vi "D_Array_to_Window.vi"(7 "Window Number (0...15)":i32, 8 "error in (no error)":errorcluster, 11 "Image Pixels (U8)":u8[][](array[numeric])) -> (0 "error out":errorcluster)   [LabVIEW 2015]
uses:
  SLM_Control_VI_source/Image_Control.dll
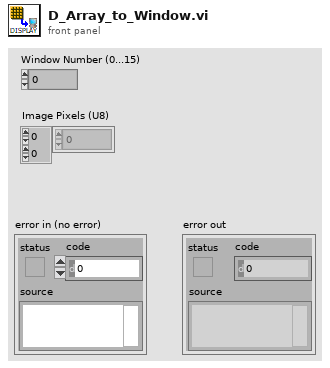
[diagram p1: front panel]
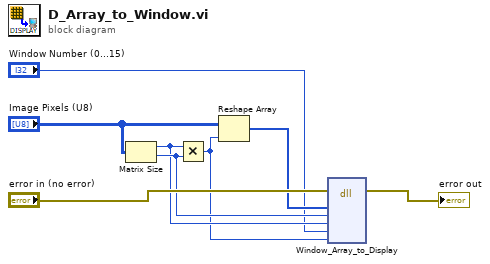
[diagram p0: block diagram]
diagram:
  n1 = Matrix Size(0:"Image Pixels (U8)") -> (1:w4:i32, 2:w5:i32)
  n2 = Multiply(x=w4, y=w5) -> (x*y=w1:i32)
  n3 = Reshape Array("Image Pixels (U8)", w1) -> (w6:u8[])
  n4 = dll-call lib="C:/Users/hs5921/Desktop/SLM_Control_VI_source/Image_Control.dll" fn="Window_Array_to_Display"(error in="error in (no error)", "1DArrayIn"=w6, "X_pixel_in"=w5, "Y_pixel_in"=w4, "WindowNum0-15"="Window Number (0...15)", "targetDataSize"=w1) -> (error out=→"error out":errorcluster)  [unwired: 8 in, 1 out]
